vi "Update State.vi"(8 "error in (no error)":errorcluster, 10 "Open?":bool, 11 "Binary Valve in":refnum<class "Binary Valve.lvclass">) -> (0 "error out":errorcluster, 3 "Binary Valve out":refnum<class "Binary Valve.lvclass">)   [LabVIEW 2021, in "Binary Valve.lvlib" / "Binary Valve.lvclass"]
uses:
  Binary Valve.lvclass
  Binary Valve.lvclass/Binary Valve.ctl
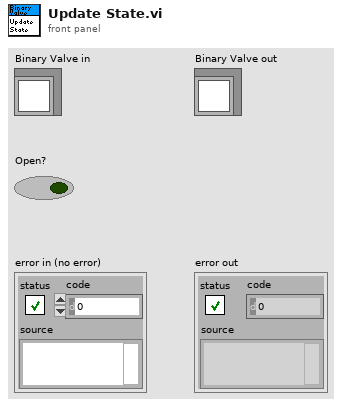
[diagram p1: front panel]
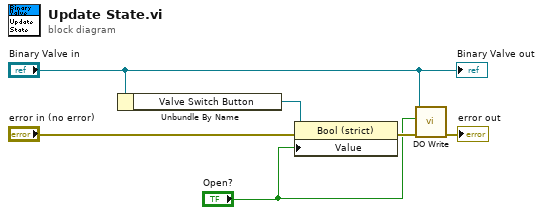
[diagram p0: block diagram]
diagram:
  n1 = Unbundle By Name("Binary Valve in") -> ("Valve Switch Button"=w6:refnum<vi>)
  n2 = property class="Bool (strict)"(reference=w6, error in="error in (no error)", "Value"="Open?") -> (error out=w5:errorcluster)  [unwired: 1 out]
  n3 = call "DO Write.vi"("error in (no error)"=w5, "Digital Output"="Open?", "Binary Valve in"="Binary Valve in") -> ("error out"=→"error out":errorcluster)  [unwired: 8 in]
  "Binary Valve out" <- "Binary Valve in"
